vi "Errors.vi"   [LabVIEW 2019, in "DSF Core.lvlib" / "Timing.lvclass"]
uses:
  Timing.lvclass
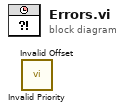
[diagram p0: block diagram]
diagram:
  n1 = call "Invalid Priority.vi"() -> ()  [unwired: 10 in, 2 out]
  n2 = call "Invalid Offset.vi"() -> ()  [unwired: 10 in, 2 out]
